vi "data combine.vi"() -> ()   [LabVIEW 2012]
uses:
  <vilib>/Utility/file.llb/Write To Spreadsheet File (DBL).vi
  <vilib>/Utility/file.llb/Read From Spreadsheet File (DBL).vi
panel:
  in  "Boolean":bool=TRUE
  in  "folder path":string="C:\\Documents and Settings\\User\\Desktop\\zw\\temp"
  out "Array":dbl[][](array[numeric])
  in  "Numeric":i32
  # "Coeff"
  # "Comm"
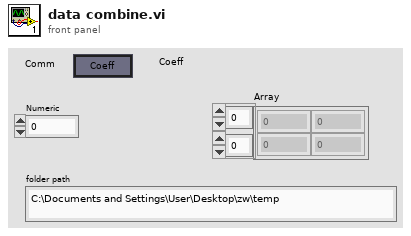
[diagram p1: front panel]
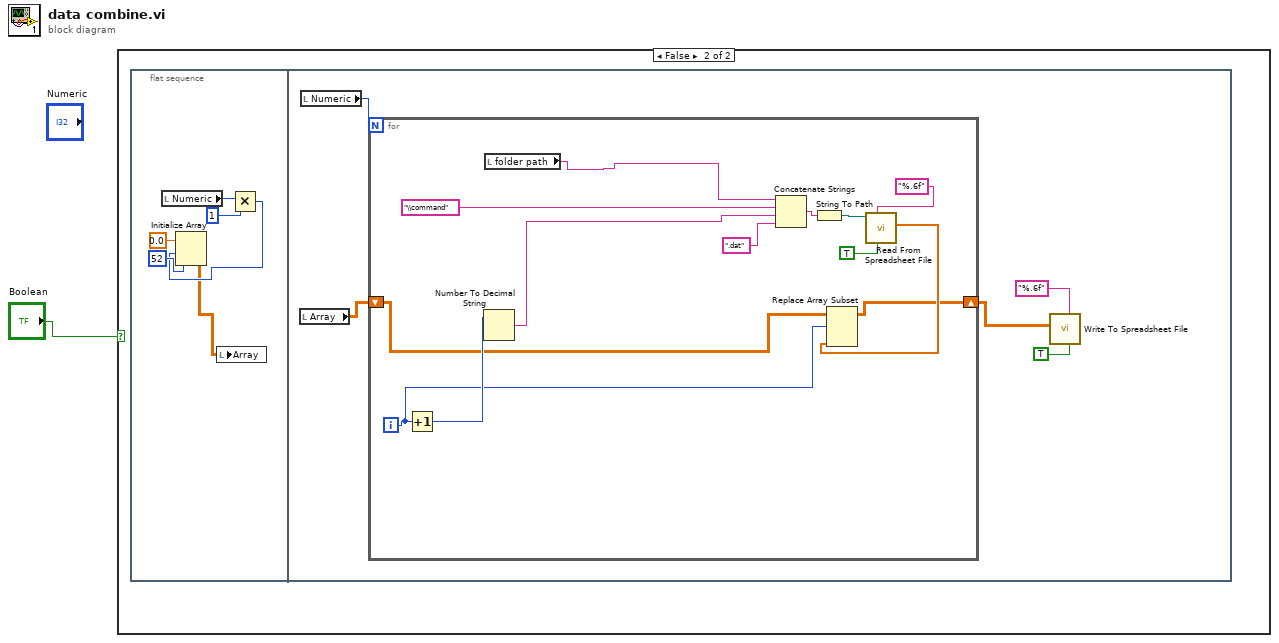
[diagram p0: block diagram]
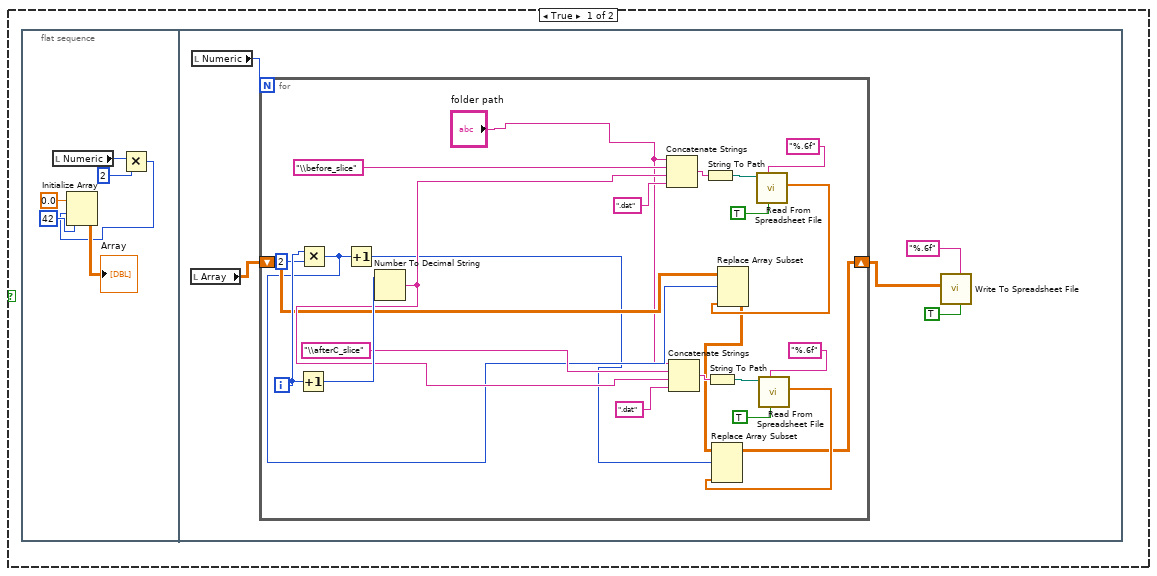
[diagram p2: hidden frame]
diagram:
  n1 = case shown="False" "Boolean" {
    frame True {
      n2 = flat-sequence {
        frame #0 {
          n3 = local read "Numeric"() -> (w4:i32)
          n4 = Multiply(x=w4, y=2) -> (x*y=w2:i32)
          n5 = Initialize Array(0.0 ("element"), w2, 42 ("dimension size")) -> (→"Array":dbl[][])
        }
        frame #1 {
          n6 = local read "Array"() -> (w9:dbl[][])
          n7 = local read "Numeric"() -> (w12:i32)
          n8 = for {
            N: w12 -> [_]
            shift-right: [w16] -> w8
            shift-left: w9 -> [w18]
            i -> [w22]
            n9 = Increment(x=w22) -> (x+1=w31:i32)
            n10 = Multiply(x=w22, y=2) -> (x*y=w15:i32)
            n11 = Increment(x=w15) -> (x+1=w14:i32)
            n12 = Number To Decimal String(number=w31) -> (decimal integer string=w20:string)  [unwired: 1 in]
            n13 = Concatenate Strings("folder path", "\\before_slice", w20, ".dat") -> (w35:string)
            n14 = Concatenate Strings("folder path", "\\afterC_slice", w20, ".dat") -> (w27:string)
            n15 = String To Path(string=w35) -> (path=w33:path)
            n16 = String To Path(string=w27) -> (path=w25:path)
            n17 = call-poly <vilib>:"Read From Spreadsheet File.vi"("transpose (no:F)"=TRUE, "format (%.3f)"="%.6f", "file path (dialog if empty)"=w33) -> ("first row"=w29:dbl[])  [unwired: 4 in, 4 out]
            n18 = Replace Array Subset(array=w18, new element=w29, index (row)=w15) -> (w19:dbl[][])  [unwired: 1 in]
            n19 = call-poly <vilib>:"Read From Spreadsheet File.vi"("transpose (no:F)"=TRUE, "format (%.3f)"="%.6f", "file path (dialog if empty)"=w25) -> ("first row"=w17:dbl[])  [unwired: 4 in, 4 out]
            n20 = Replace Array Subset(array=w19, new element=w17, index (row)=w14) -> (w16:dbl[][])  [unwired: 1 in]
          }
          n21 = call-poly <vilib>:"Write To Spreadsheet File.vi"("transpose? (no:F)"=TRUE, "format (%.3f)"="%.6f", "2D data"=w8) -> ()  [unwired: 5 in, 1 out]
        }
      }
    }
    frame False {
      n22 = flat-sequence {
        frame #0 {
          n23 = local read "Numeric"() -> (w40:i32)
          n24 = Multiply(x=w40, y=1) -> (x*y=w38:i32)
          n25 = Initialize Array(0.0 ("element"), w38, 52 ("dimension size")) -> (w37:dbl[][])
          n26 = local write "Array"(w37) -> ()
        }
        frame #1 {
          n27 = local read "Array"() -> (w44:dbl[][])
          n28 = local read "Numeric"() -> (w47:i32)
          n29 = for {
            N: w47 -> [_]
            shift-right: [w48] -> w43
            shift-left: w44 -> [w51]
            i -> [w49]
            n30 = Increment(x=w49) -> (x+1=w55:i32)
            n31 = Number To Decimal String(number=w55) -> (decimal integer string=w52:string)  [unwired: 1 in]
            n32 = local read "folder path"() -> (w50:string)
            n33 = Concatenate Strings(w50, "\\command", w52, ".dat") -> (w59:string)
            n34 = String To Path(string=w59) -> (path=w57:path)
            n35 = call-poly <vilib>:"Read From Spreadsheet File.vi"("transpose (no:F)"=TRUE, "format (%.3f)"="%.6f", "file path (dialog if empty)"=w57) -> ("first row"=w53:dbl[])  [unwired: 4 in, 4 out]
            n36 = Replace Array Subset(array=w51, new element=w53, index (row)=w49) -> (w48:dbl[][])  [unwired: 1 in]
          }
          n37 = call-poly <vilib>:"Write To Spreadsheet File.vi"("transpose? (no:F)"=TRUE, "format (%.3f)"="%.6f", "2D data"=w43) -> ()  [unwired: 5 in, 1 out]
        }
      }
    }
  }
